vi "Write Patch.vi"(8 "error in (no error)":errorcluster, 10 "Patch":i32, 11 "Semver in":refnum<class "Semver.lvclass">) -> (0 "error out":errorcluster, 3 "Semver out":refnum<class "Semver.lvclass">)   [LabVIEW 2017, in "Semver.lvlib" / "Semver.lvclass"]
uses:
  Semver.lvclass
  Semver.lvclass/Semver.ctl
  <vilib>/Utility/error.llb/Error Cluster From Error Code.vi
  <vilib>/ErrorRing/Error Ring.xnode
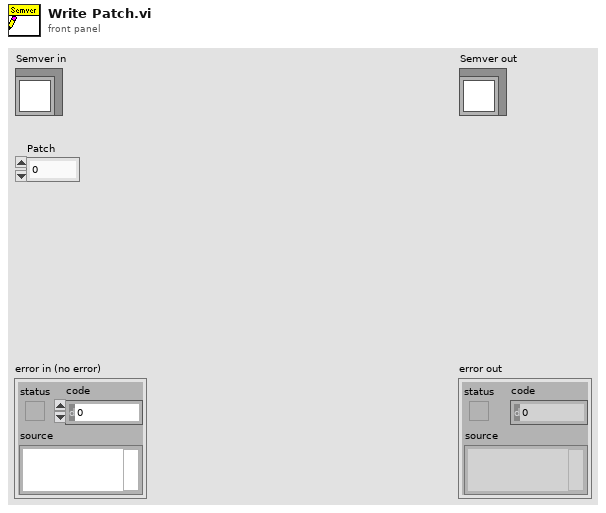
[diagram p1: front panel]
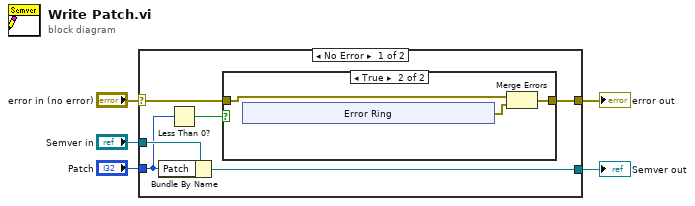
[diagram p0: block diagram]
diagram:
  n1 = case shown="No Error" "error in (no error)" {
    selector: "error in (no error)" -> [w9 w21]
    tunnel: [w8 w21] -> w4
    tunnel: [w10 w22] -> w2
    tunnel: "Semver in" -> [w11 w22]
    tunnel: "Patch" -> [w7 _]
    frame No Error {
      n2 = Bundle By Name(cluster=w11, "Patch"=w7) -> (w10:refnum<class "Semver.lvclass">)
      n3 = Less Than 0?(x=w7) -> (x < 0?=w6:bool)
      n4 = case shown="True" w6 {
        tunnel: w9 -> [w12 w15]
        tunnel: [w12 w14] -> w8
        frame False {
        }
        frame True {
          n5 = xnode "Error Ring"() -> ("error out"=w13:errorcluster)
          n6 = Merge Errors(w15, w13) -> (w14:errorcluster)
        }
      }
    }
    frame Error {
    }
  }
  "error out" <- w4
  "Semver out" <- w2
